vi "OpenLog.vi"(8 "error in (no error)":errorcluster, 9 "DUTIndex":i32, 10 "TimeString":string, 11 "Directory":string="D:\\MitraStar\\New Solution\\Teststand\\SubVI") -> (0 "error out":errorcluster, 3 "refnum out":refnum<file>)   [LabVIEW 2012]
panel:
  out "path":path=path "D:/.txt"
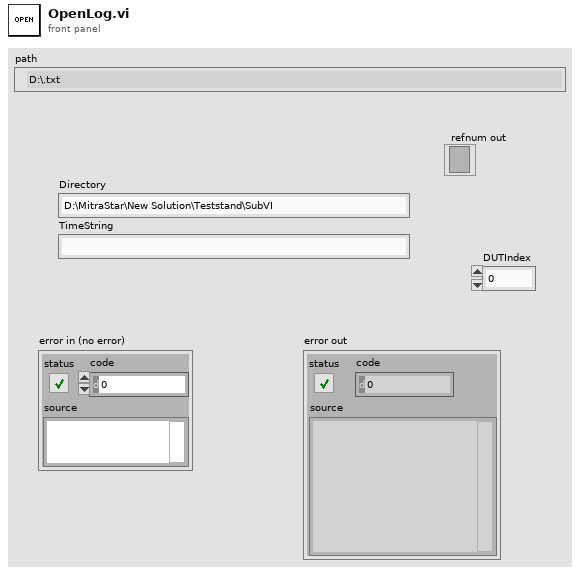
[diagram p1: front panel]
types:
  T1 = enum16{"open", "replace", "create", "open or create", "replace or create", "replace or create with confirmation"}
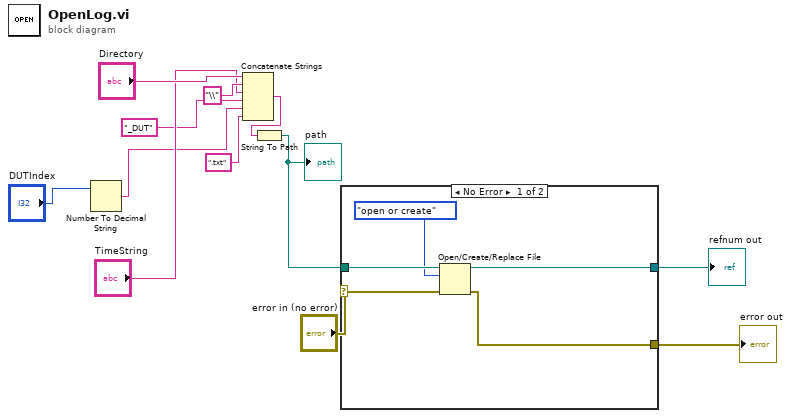
[diagram p0: block diagram]
diagram:
  n1 = Number To Decimal String(number="DUTIndex") -> (decimal integer string=w1:string)  [unwired: 1 in]
  n2 = Concatenate Strings("Directory", "\\" ("string"), "TimeString", "_DUT" ("string"), w1, ".txt" ("string")) -> (w7:string)
  n3 = String To Path(string=w7) -> (path=w9:path)
  "path" <- w9
  n4 = case shown="No Error" "error in (no error)" {
    selector: "error in (no error)" -> [w16 w18]
    tunnel: w9 -> [w17 _]
    tunnel: [w15 w18] -> w11
    tunnel: [w14 _] -> w10
    frame No Error {
      n5 = Open/Create/Replace File(file path (use dialog)=w17, error in=w16, operation (0:open)=T1."open or create") -> (refnum out=w14:refnum<file>, error out=w15:errorcluster)  [unwired: 3 in, 1 out]
    }
    frame Error {
    }
  }
  "error out" <- w11
  "refnum out" <- w10
